vi "__uintSetBaseUintTimeout.vi"(7 "Uint in":u8[](array[numeric]), 8 "Error in (no error)":errorcluster, 9 "Base (decimal)":T2 items=["Binary"=2, "Octal"=8, "Decimal"=10, "Hexadecimal"=16, "Hexatrigesimal"=36, "ASCII"=64], 10 "Timeout (-1)":T1, 11 "UintClass in":refnum<class "UintClass.lvclass">) -> (0 "Error out":errorcluster, 3 "UintClass out":refnum<class "UintClass.lvclass">)   [LabVIEW 2011, in "UintClass.lvclass"]
uses:
  UintClass.lvclass
  enumBase.ctl
  timeout.ctl
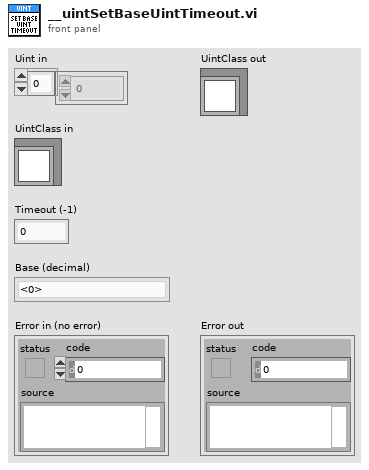
[diagram p1: front panel]
types:
  T1 = typedef "UintClass.lvclass/timeout.ctl" = i32
  T2 = typedef "UintClass.lvclass/enumBase.ctl" = u16
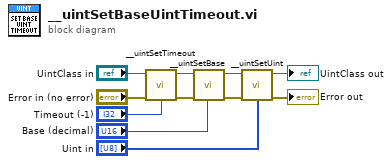
[diagram p0: block diagram]
diagram:
  n1 = call "__uintSetTimeout.vi"("Error in (no error)"="Error in (no error)", "Timeout (-1)"="Timeout (-1)", "Uint in"="UintClass in") -> ("Error out"=w5:errorcluster, "Uint out"=w4:refnum<class "UintClass.lvclass">)  [unwired: 7 in]
  n2 = call "__uintSetBase.vi"("Error in (no error)"=w5, "Base (decimal)"="Base (decimal)", "Uint in"=w4) -> ("Error out"=w7:errorcluster, "Uint out"=w6:refnum<class "UintClass.lvclass">)  [unwired: 7 in]
  n3 = call "__uintSetUint.vi"("Error in (no error)"=w7, 10:"Uint in"="Uint in", 11:"Uint in"=w6) -> ("Error out"=→"Error out":errorcluster, "Uint out"=→"UintClass out":refnum<class "UintClass.lvclass">)  [unwired: 7 in]
